vi "Tipstrip Mouse Leave (XY Graph).vi"(7 "TipStrip Refnum":refnum<vi>, 8 "Error In":errorcluster, 10 "Event Registration Refnum in":refnum<event-registration>, 11 "XYGraph Refnum":refnum<vi>) -> (0 "Error Out":errorcluster, 2 "Event Registration Refnum out":refnum<event-registration>)   [LabVIEW 2021, in "XY Graph Add-Ons.lvlib"]
doc: "Connect the corresponding dynamic event clusters of the Event Structure's \"Mouse Leave\" event for the XYGraph to this subVI"
uses:
  XY Graph/XY Graph Add-Ons.lvlib
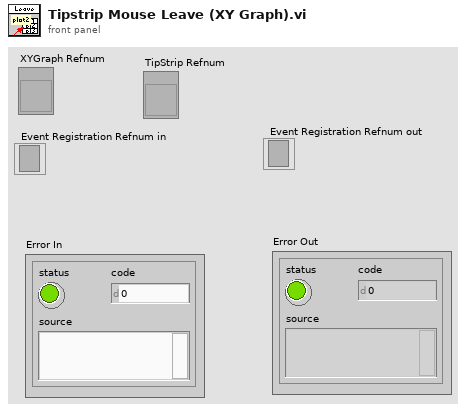
[diagram p1: front panel]
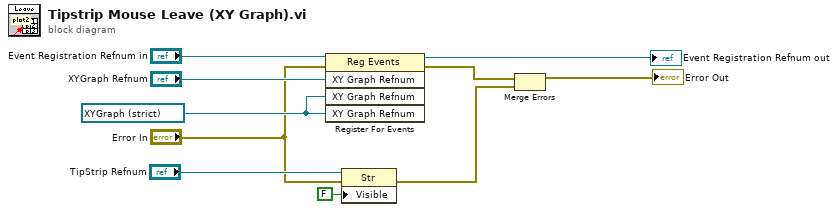
[diagram p0: block diagram]
diagram:
  w8 = refnum<vi> refnum ("event source")
  n1 = register-events(reference="Event Registration Refnum in", error in="Error In", "XYGraph Refnum", w8, w8) -> (reference out=→"Event Registration Refnum out":refnum<event-registration>, error out=w2:errorcluster)
  n2 = property class="Str"(reference="TipStrip Refnum", error in="Error In", "Visible"=FALSE) -> (error out=w1:errorcluster)  [unwired: 1 out]
  n3 = Merge Errors(w2, w1) -> (→"Error Out":errorcluster)
